vi "modbus slave new.vi"() -> ()   [LabVIEW 2016]
uses:
  <vilib>/NI/Modbus Library/API/Wrapper/Create TCP Slave.vi
  <vilib>/NI/Modbus Library/API/Slave/Modbus Slave.lvclass
  <vilib>/NI/Modbus Library/API/Wrapper/API Main.lvlib
  <vilib>/ptbypt/NI_PtbyPt.lvlib
panel:
  out "读取register values 2":u16[](array[numeric])
  out "status":bool
  in  "写入registers to write":u16[](array[numeric])
  out "读取register values":u16[](array[numeric])
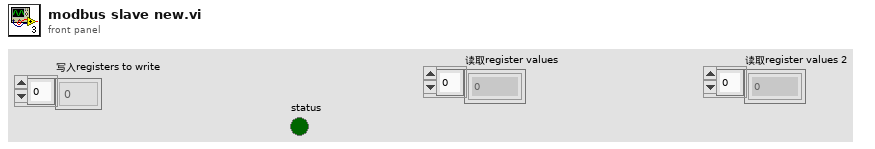
[diagram p1: front panel]
types:
  T1 = enum16{"", "CODMn", "PH", "氨氮", "总氮", "总磷", "CODCr", "电导率", "水温", "溶解氧", "浊度", "叶绿素", "藻密度", "ORP"}
  T2 = enum16{"i13001", "i13002", "i13003", "i13004", "i13005", "i13006", "i13007", "i13008", "i13009", "i13010", "i13011", "i13012", "i13013", "i13014", "i13015", "i13016", "i13017", "i13101", "i13102", "i13103", "i13104", "i13105", "i13106", "i13107", "i13108", "i13109", "i13110"}
  T3 = enum16{"启动整机", "停止整机", "标样核查", "加标回收", "平行样测试", "零点核查", "跨度核查", "校零", "校标"}
  T4 = cluster{"status":bool, "代码":u16, "source":string}
  T5 = cluster{"COD浓度（mg/L)":dbl, "水样启动时间":timestamp, "加标回收启动时间":timestamp, "CODMn工作状态":enum16{"空闲", "水样测试", "标样核查", "零点核查", "跨度核查", "空白测试", "平行样测试", "加标回收", "空白校准", "标样校准", "初始化（清洗）"}, "多列列表框":i32}
  T6 = cluster{"系统时间":timestamp, "工作状态":enum16{"空闲", "水样测试", "标样核查", "零点核查", "跨度核查", "空白测试", "平行样测试", "加标回收", "空白校准", "标样校准", "初始化（清洗）"}, "测量模式":enum16{"待机", "连续模式", "周期模式", "定点模式", "受控模式", "手动模式"}, "告警代码":u16, "故障代码":u16, "日志代码":u16, "软件版本":u16, "F0":sgl, "F1":sgl, "F2":sgl, "F3":sgl, "T":sgl, "H":sgl, "id":u16, "flowid":u16, "量程":u16, "总磷控温温度1":sgl, "营养盐控温温度2":sgl, "ADC":sgl}
  T7 = enum16{"空闲", "水样测试", "标样核查", "零点核查", "跨度核查", "空白测试", "平行样测试", "加标回收", "空白校准", "标样校准", "初始化（清洗）"}
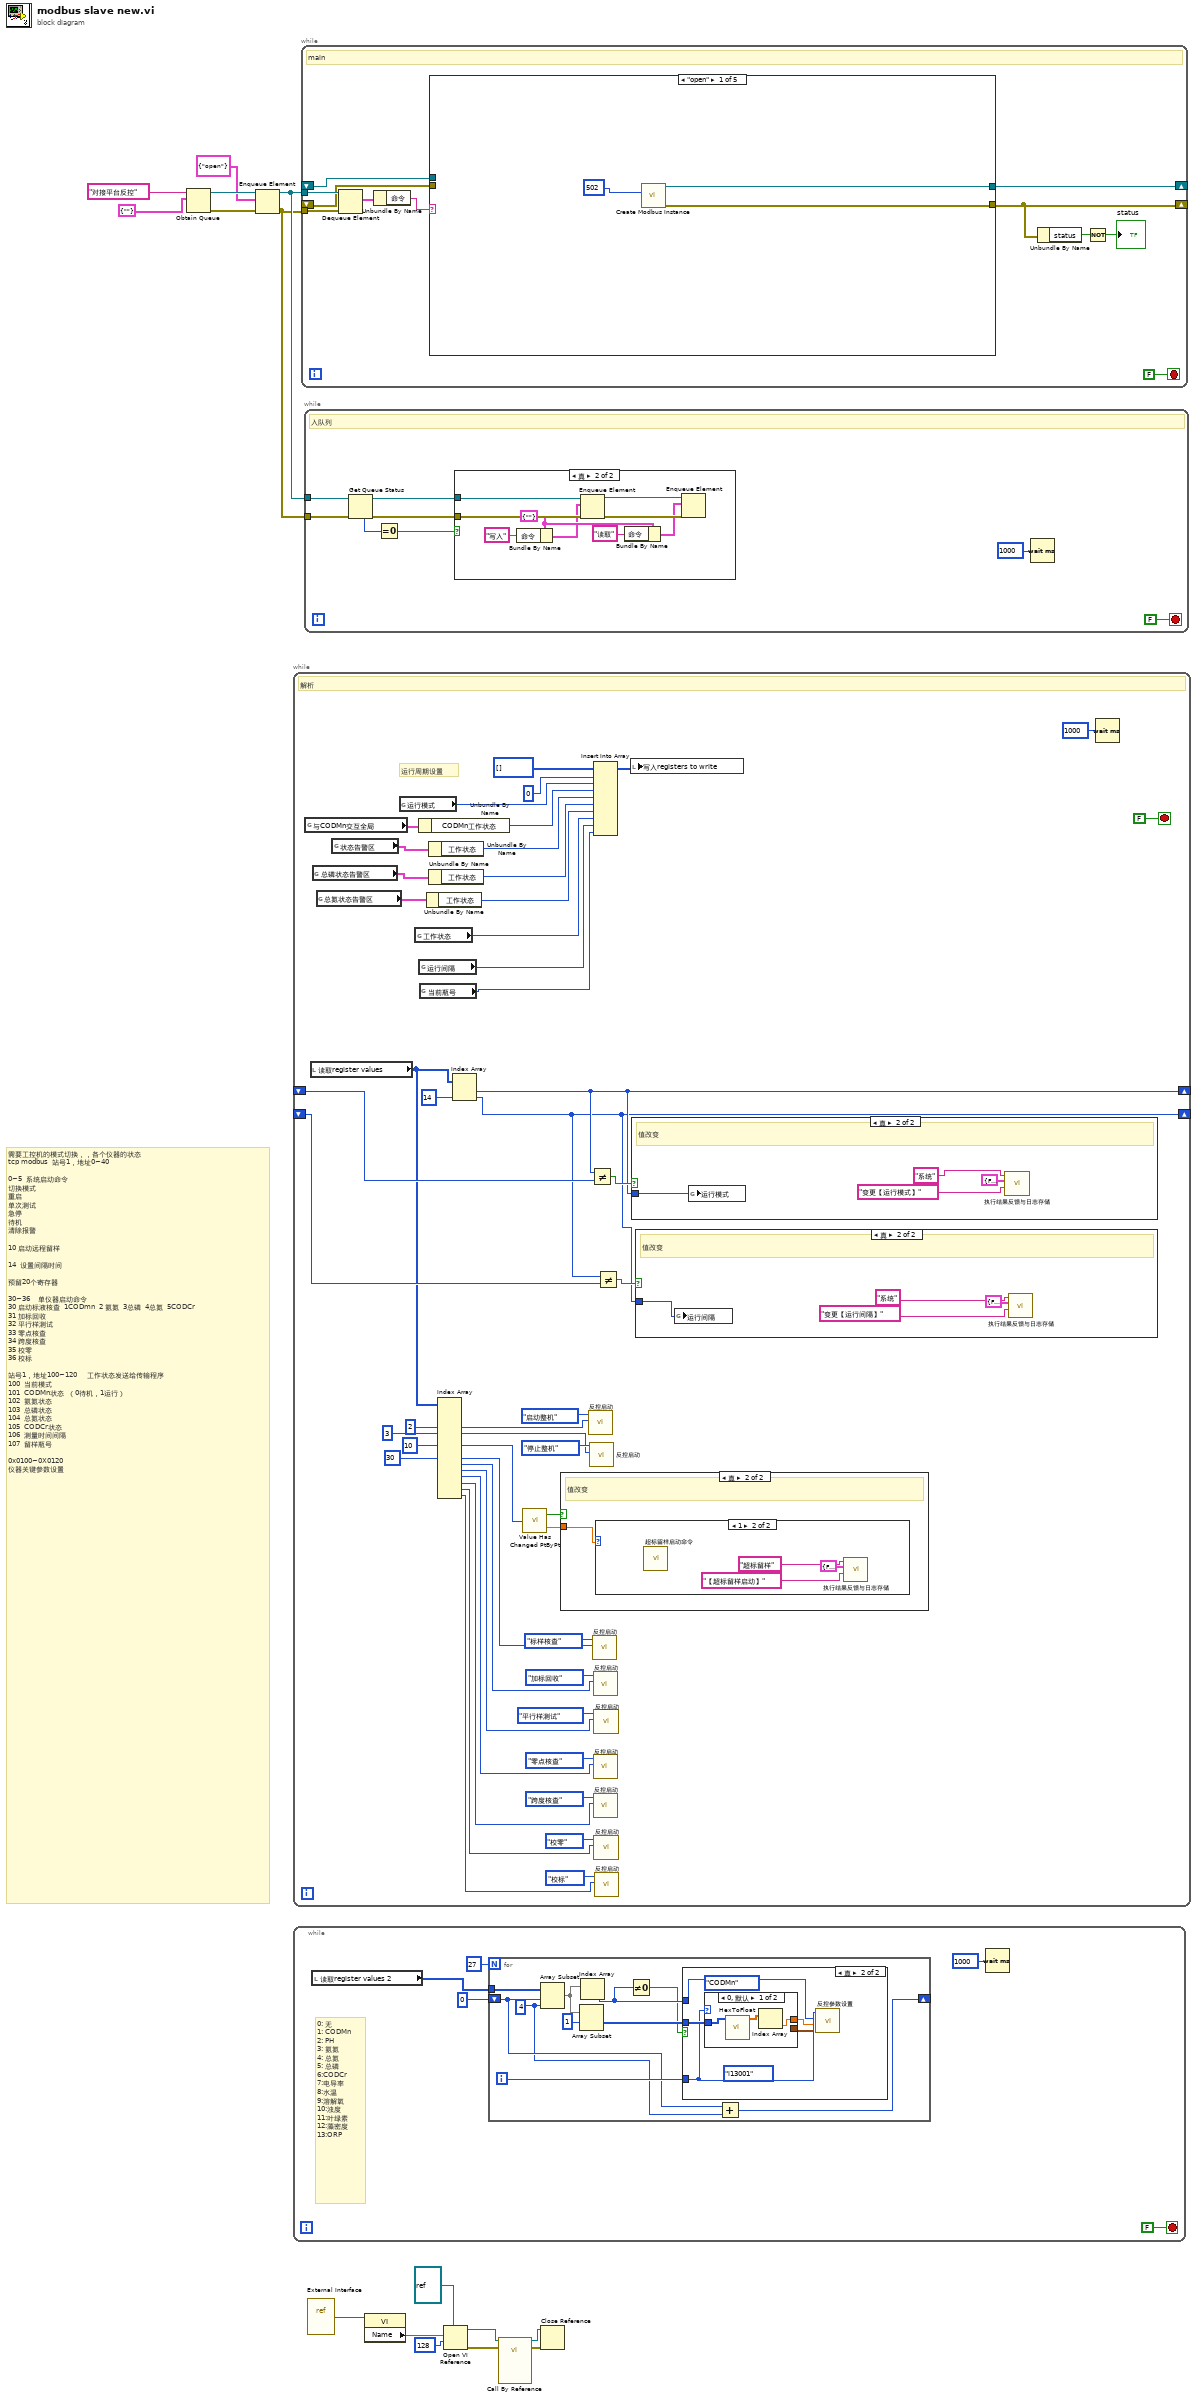
[diagram p0: block diagram]
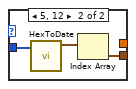
[diagram p3: hidden frame]
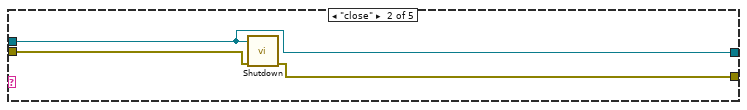
[diagram p9: hidden frame]
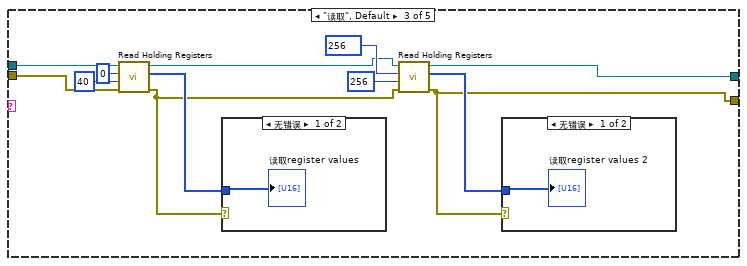
[diagram p10: hidden frame]
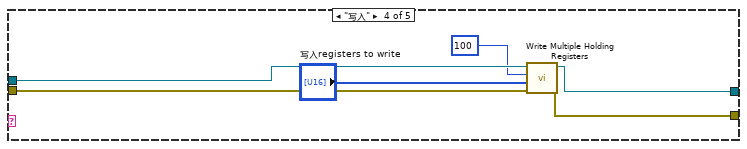
[diagram p13: hidden frame]
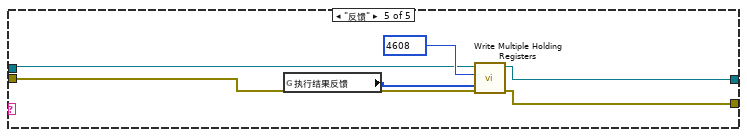
[diagram p14: hidden frame]
diagram:
  # "需要工控机的模式切换，，各个仪器的状态\ntcp modbus  站号1，地址0~40\n\n0~5  系统启动命令\n切换模式\n重启\n单次测试\n急停\n待机\n清除报警\n\n10 启动远程留样\n\n14  设置间隔时间\n\n预留20个寄存器\n\n30~36    单仪器启动命令\n30 启动标液核查  1CODmn  2 氨氮  3总磷  4总氮  5CODCr\n31 加标回收\n32 平行样测试\n33 零点核查\n34 跨度核查\n35 校零\n36 校标\n\n站号1，地址100~120     工作状态发送给传输程序\n100  当前模式\n101  CODMn状态  （0待机，1运行）\n102  氨氮状态\n103  总磷状态\n104  总氮状态\n105  CODCr状态\n106  测量时间间隔\n107  留样瓶号\n\n0x0100~0X0120\n仪器关键参数设置"
  n1 = Obtain Queue(name (unnamed)="对接平台反控" ("名称（未命名）"), element data type=cluster{"命令":string} {"命令"=""}) -> (queue out=w13:refnum<queue>, error out=w12:errorcluster)  [unwired: 3 in, 1 out]
  n2 = Enqueue Element(queue=w13, element=cluster{"命令":string} {"命令"="open"} ("元素"), error in (no error)=w12) -> (queue out=w10:refnum<queue>, error out=w9:errorcluster)  [unwired: 1 in, 1 out]
  n3 = while {
    stop <- FALSE stop-if-true
    # "0: 无\n1: CODMn\n2: PH\n3: 氨氮\n4: 总氮\n5: 总磷\n6:CODCr\n7:电导率\n8:水温\n9:溶解氧\n10:浊度\n11:叶绿素\n12:藻密度\n13:ORP"
    n4 = local read "读取register values 2"() -> (w18:u16[])
    n5 = for {
      N: 27 -> [_]
      tunnel: w18 -> [w30]
      shift-right: [w21] -> _
      shift-left: 0 ("索引") -> [w23]
      i -> [w26]
      w22 = 4 ("长度")
      n6 = Array Subset(array=w30, index=w23, length=w22) -> (w29:u16[])
      n7 = Array Subset(array=w29, index=1 ("索引")) -> (w27:u16[])  [unwired: 1 in]
      n8 = Index Array(array=w29) -> (element=w25:u16)  [unwired: 1 in]
      n9 = Not Equal To 0?(x=w25) -> (x != 0?=w24:bool)
      n10 = case shown="真" w24 {
        tunnel: w27 -> [_ w35]
        tunnel: w26 -> [_ w34]
        tunnel: w25 -> [_ w33]
        frame False {
        }
        frame True {
          (unwired) T1."CODMn"
          (unwired) T2."i13001" ("设置类型")
          n11 = case shown="0, 默认" w34 {
            tunnel: w35 -> [w37 w40]
            tunnel: [_ w41] -> w31
            tunnel: [w38 _] -> w32
            frame 0, Default {
              n12 = call "HexToFloat.vi"("数组"=w37) -> ("FLOAT"=w36:sgl[])  [unwired: 10 in]
              n13 = Index Array(array=w36) -> (element=w38:sgl)  [unwired: 1 in]
            }
            frame 5, 12 {
              n14 = call "HexToDate.vi"("数组"=w40) -> ("DATE"=w39:timestamp[])  [unwired: 10 in]
              n15 = Index Array(array=w39) -> (element=w41:timestamp)  [unwired: 1 in]
            }
          }
          n16 = call "反控参数设置.vi"("value time"=w31, "value float"=w32, "设置参数"=w33, "设置类型"=w34) -> ()  [unwired: 8 in]
        }
      }
      n17 = Add(x=w23, y=w22) -> (x+y=w21:i32)
    }
    n18 = Wait (ms)(milliseconds to wait=u32 1000 ("等待时间（毫秒）")) -> ()  [unwired: 1 out]
  }
  n19 = while {
    shift-right: [w77] -> _
    shift-left: _ -> [w79]
    shift-right: [w74] -> _
    shift-left: _ -> [w76]
    stop <- FALSE stop-if-true
    # "运行周期设置"
    # "解析"
    n20 = global read "modbus slave全局.vi" "与CODMn交互全局"() -> (w46:T5)
    n21 = local read "读取register values"() -> (w69:u16[])
    n22 = global read "VAR总磷总氮全局变量.vi" "总磷状态告警区"() -> (w43:T6)
    n23 = global read "VAR总磷总氮全局变量.vi" "总氮状态告警区"() -> (w42:T6)
    n24 = global read "VAR氨氮全局变量.vi" "状态告警区"() -> (w44:T6)
    n25 = global read "系统设置全局变量.vi" "运行模式"() -> (w88:enum16{"维护模式", "常规模式", "应急模式", "质控模式"})
    n26 = global read "CODcr全局变量.vi" "工作状态"() -> (w83:T7)
    n27 = Unbundle By Name(w46) -> ("CODMn工作状态"=w45:T7)
    n28 = global read "系统设置全局变量.vi" "运行间隔"() -> (w82:i16)
    n29 = global read "外部交互全局.vi" "当前瓶号"() -> (w47:u16)
    n30 = Unbundle By Name(w42) -> ("工作状态"=w84:T7)
    n31 = Unbundle By Name(w44) -> ("工作状态"=w86:T7)
    n32 = Unbundle By Name(w43) -> ("工作状态"=w85:T7)
    n33 = Index Array(array=w69, index #3=2 ("索引"), index #4=3 ("索引"), index #6=10 ("索引"), index #8=30 ("索引")) -> (element #3=w68:u16, element #4=w65:u16, element #6=w62:u16, element #8=w60:u16, element #9=w54:u16, element #10=w53:u16, element #11=w52:u16, element #12=w50:u16, element #13=w49:u16, element #14=w48:u16)  [unwired: 10 in, 4 out]
    n34 = Index Array(array=w69, index #2=14 ("索引")) -> (element #1=w77:u16, element #2=w74:u16)  [unwired: 1 in]
    n35 = call <vilib>:"Value Has Changed PtByPt.vi"("input data point"=w62) -> ("has changed"=w64:bool, "output data point"=w63:dbl)  [unwired: 1 in]
    n36 = case shown="真" w64 {
      tunnel: w63 -> [_ w92]
      frame False {
      }
      frame True {
        # "值改变"
        n37 = case shown="1" w92 {
          frame 0, Default {
          }
          frame 1 {
            n38 = call "超标留样启动命令.vi"() -> ()  [unwired: 12 in]
            n39 = call "执行结果反馈与日志存储.vi"("日志信息"="【超标留样启动】", "error out"=T4 {"status"=FALSE, "代码"=1, "source"=""}, "设备"="超标留样") -> ()  [unwired: 9 in]
          }
        }
      }
    }
    n40 = call "反控启动.vi"("启动参数"=w68, "启动类型"=T3."启动整机") -> ()  [unwired: 10 in]
    n41 = call "反控启动.vi"("启动参数"=w65, "启动类型"=T3."停止整机") -> ()  [unwired: 10 in]
    n42 = Not Equal?(x=w77, y=w79) -> (x != y?=w78:bool)
    n43 = call "反控启动.vi"("启动参数"=w60, "启动类型"=T3."标样核查") -> ()  [unwired: 10 in]
    n44 = Insert Into Array(array=u16[] [] ("values to write"), index=0 ("索引"), new element #1=w88, new element #2=w45, new element #3=w86, new element #4=w85, new element #5=w84, new element #6=w83, new element #7=w82, new element #8=w47) -> (w81:u16[])
    n45 = call "反控启动.vi"("启动参数"=w54, "启动类型"=T3."加标回收") -> ()  [unwired: 10 in]
    n46 = call "反控启动.vi"("启动参数"=w52, "启动类型"=T3."零点核查") -> ()  [unwired: 10 in]
    n47 = call "反控启动.vi"("启动参数"=w50, "启动类型"=T3."跨度核查") -> ()  [unwired: 10 in]
    n48 = call "反控启动.vi"("启动参数"=w53, "启动类型"=T3."平行样测试") -> ()  [unwired: 10 in]
    n49 = call "反控启动.vi"("启动参数"=w49, "启动类型"=T3."校零") -> ()  [unwired: 10 in]
    n50 = call "反控启动.vi"("启动参数"=w48, "启动类型"=T3."校标") -> ()  [unwired: 10 in]
    n51 = Not Equal?(x=w74, y=w76) -> (x != y?=w75:bool)
    n52 = local write "写入registers to write"(w81) -> ()
    n53 = case shown="真" w78 {
      tunnel: w77 -> [_ w103]
      frame False {
      }
      frame True {
        # "值改变"
        n54 = global write "系统设置全局变量.vi" "运行模式"(w103) -> ()
        n55 = call "执行结果反馈与日志存储.vi"("日志信息"="变更【运行模式】", "error out"=T4 {"status"=FALSE, "代码"=1, "source"=""}, "设备"="系统") -> ()  [unwired: 9 in]
      }
    }
    n56 = case shown="真" w75 {
      tunnel: w74 -> [_ w99]
      frame False {
      }
      frame True {
        # "值改变"
        n57 = global write "系统设置全局变量.vi" "运行间隔"(w99) -> ()
        n58 = call "执行结果反馈与日志存储.vi"("日志信息"="变更【运行间隔】", "error out"=T4 {"status"=FALSE, "代码"=1, "source"=""}, "设备"="系统") -> ()  [unwired: 9 in]
      }
    }
    n59 = Wait (ms)(milliseconds to wait=u32 1000 ("等待时间（毫秒）")) -> ()  [unwired: 1 out]
  }
  n60 = while {
    tunnel: w10 -> [w114]
    tunnel: w9 -> [w113]
    shift-right: [w110] -> _
    shift-left: _ -> [w109]
    shift-right: [w104] -> _
    shift-left: _ -> [w108]
    stop <- FALSE stop-if-true
    # "main"
    n61 = Dequeue Element(queue=w114, error in (no error)=w113) -> (element=w112:cluster{"命令":string})  [unwired: 1 in, 3 out]
    n62 = Unbundle By Name(w112) -> ("命令"=w111:string)
    n63 = case shown="\"open\"" w111 {
      tunnel: [w115 w118 w122 w136 w143] -> w110
      tunnel: [w116 w119 w121 w135 w142] -> w104
      tunnel: w109 -> [_ w118 w132 w140 w145]
      tunnel: w108 -> [_ w120 w131 w139 w144]
      frame "open" {
        n64 = call-poly <vilib>:"Create Modbus Instance.vi"("port (502)"=u16 502) -> ("error out"=w116:errorcluster, "TCP slave instance"=w115:refnum<class "Modbus Slave.lvclass">)  [unwired: 9 in]
      }
      frame "close" {
        n65 = call-dynamic "Shutdown.vi"("error in"=w120, "Modbus slave in"=w118) -> ("error out"=w119:errorcluster)  [unwired: 9 in]
      }
      frame "读取", Default {
        n66 = call-dynamic "Read Holding Registers.vi"("error in"=w131, "number of inputs"=u16 40, "starting address"=u16 0, "Modbus slave in"=w132) -> ("error out"=w123:errorcluster, "register values"=w128:u16[], "Modbus slave out"=w124:refnum<class "Modbus Slave.lvclass">)  [unwired: 5 in]
        n67 = case shown="无错误" w123 {
          tunnel: w128 -> [w134 _]
          frame No Error {
            "读取register values" <- w134
          }
          frame Error {
          }
        }
        n68 = call-dynamic "Read Holding Registers.vi"("error in"=w123, "number of inputs"=u16 256, "starting address"=u16 256, "Modbus slave in"=w124) -> ("error out"=w121:errorcluster, "register values"=w127:u16[], "Modbus slave out"=w122:refnum<class "Modbus Slave.lvclass">)  [unwired: 5 in]
        n69 = case shown="无错误" w121 {
          tunnel: w127 -> [w133 _]
          frame No Error {
            "读取register values 2" <- w133
          }
          frame Error {
          }
        }
      }
      frame "写入" {
        n70 = call-dynamic "Write Multiple Holding Registers.vi"("error in"=w139, "registers to write"="写入registers to write", "starting address"=u16 100, "Modbus slave in"=w140) -> ("error out"=w135:errorcluster, "Modbus slave out"=w136:refnum<class "Modbus Slave.lvclass">)  [unwired: 6 in]
      }
      frame "反馈" {
        n71 = global read "modbus slave全局.vi" "执行结果反馈"() -> (w141:u16[])
        n72 = call-dynamic "Write Multiple Holding Registers.vi"("error in"=w144, "registers to write"=w141, "starting address"=u16 4608, "Modbus slave in"=w145) -> ("error out"=w142:errorcluster, "Modbus slave out"=w143:refnum<class "Modbus Slave.lvclass">)  [unwired: 6 in]
      }
    }
    n73 = Unbundle By Name(w104) -> ("status"=w106:bool)
    n74 = Not(x=w106) -> (.not. x?=→"status":bool)
  }
  n75 = while {
    tunnel: w10 -> [w154]
    tunnel: w9 -> [w152]
    stop <- FALSE stop-if-true
    # "入队列"
    n76 = Get Queue Status(queue=w154, error in (no error)=w152) -> (queue out=w153:refnum<queue>, error out=w151:errorcluster, # elements in queue=w150:i32)  [unwired: 1 in, 5 out]
    n77 = Equal To 0?(x=w150) -> (x = 0?=w149:bool)
    n78 = case shown="真" w149 {
      tunnel: w153 -> [_ w163]
      tunnel: w151 -> [_ w162]
      frame False {
      }
      frame True {
        w158 = cluster{"命令":string} {"命令"=""} ("元素")
        n79 = Bundle By Name(cluster=w158, "命令"="写入") -> (w157:cluster{"命令":string})
        n80 = Enqueue Element(queue=w163, element=w157, error in (no error)=w162) -> (queue out=w161:refnum<queue>, error out=w160:errorcluster)  [unwired: 1 in, 1 out]
        n81 = Bundle By Name(cluster=w158, "命令"="读取") -> (w155:cluster{"命令":string})
        n82 = Enqueue Element(queue=w161, element=w155, error in (no error)=w160) -> ()  [unwired: 1 in, 3 out]
      }
    }
    n83 = Wait (ms)(milliseconds to wait=u32 1000 ("等待时间（毫秒）")) -> ()  [unwired: 1 out]
  }
  n84 = vi-ref "External Interface.vi"() -> (w8:refnum<vi>)
  n85 = property class="VI"(reference=w8) -> ("Name"=w7:string)  [unwired: 1 in, 2 out]
  n86 = Open VI Reference(type specifier VI Refnum (for type only)=refnum<vi> refnum, vi path=w7, options=128 ("选项")) -> (vi reference=w5:refnum<vi>, error out=w3:errorcluster)  [unwired: 3 in]
  n87 = call-by-ref "?"(reference=w5, error in=w3) -> (reference out=w1:refnum<vi>, error out=w2:errorcluster)  [unwired: 12 in]
  n88 = Close Reference(reference=w1, error in (no error)=w2) -> ()  [unwired: 1 out]
